vi "I2CConfigure.vi"(7 "Address Type (7-bit)":enum16{"7-bit", "10-bit"}(ring), 8 "error in (no error)":errorcluster caption="ErrorIn", 9 "Clock Rate":u32, 10 "IICSlaveAddress":u16, 11 "FPGA VI引用输入":refnum<k20>) -> (0 "error out":errorcluster caption="ErrorOut", 3 "FPGA VI引用输出":refnum<k20>)   [LabVIEW 2015]
uses:
  <vilib>/Utility/error.llb/Error Cluster From Error Code.vi
  <vilib>/rvi/errors/niLvFpgaAdjustHostInterfaceError.vi
  <vilib>/rvi/interface/nirviReadWriteControl/nirviReadWriteControl.xnode
  IEDriver/IEDriver/SPIandI2C/FPGA/Library/IP SPI&I2C.lvlib
  NiFpgaLv.dll
  <vilib>/rvi/interface/Simulation/niFpgaSimulationCallBeginRW.vi
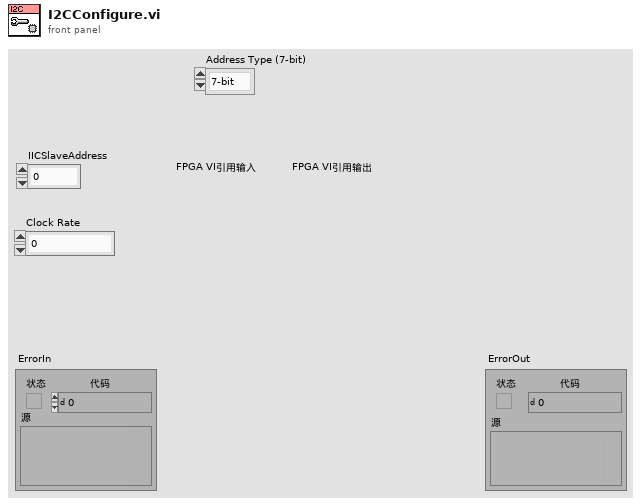
[diagram p1: front panel]
types:
  T1 = cluster{"Address Type (7-bit)":enum16{"7-bit", "10-bit"}, "IICSlaveAddress":u16, "I2C Parameters":cluster{"Clock Divider":u32}}
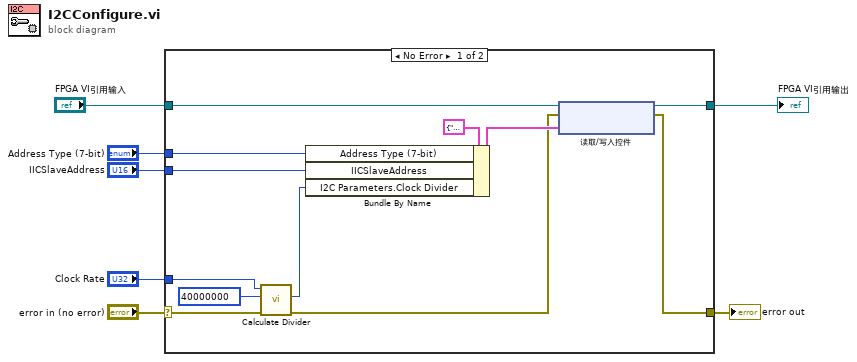
[diagram p0: block diagram]
diagram:
  n1 = case shown="No Error" "error in (no error)" {
    selector: "error in (no error)" -> [w18 w21]
    tunnel: "FPGA VI引用输入" -> [w19 w20]
    tunnel: "Clock Rate" -> [w16 _]
    tunnel: "Address Type (7-bit)" -> [w13 _]
    tunnel: "IICSlaveAddress" -> [w12 _]
    tunnel: [w9 w21] -> w3
    tunnel: [w8 w20] -> w1
    frame No Error {
      n2 = call "Calculate Divider.vi"("error in"=w18, "FPGA Clock (Hz)"=u32 40000000 ("Clock Rate (Hz)"), "Clock Rate (Hz)"=w16) -> ("error out"=w10:errorcluster, "Clock Divider"=w11:u32)  [unwired: 6 in, 1 out]
      n3 = Bundle By Name(cluster=T1 {"Address Type (7-bit)"=enum."7-bit", "IICSlaveAddress"=0, "I2C Parameters"={"Clock Divider"=0}} ("IICParameters"), "Address Type (7-bit)"=w13, "IICSlaveAddress"=w12, "I2C Parameters.Clock Divider"=w11) -> (w14:T1)
      n4 = xnode "读取/写入控件"("FPGA VI Reference In"=w19, "error in"=w10, "IICParameters"=w14) -> ("FPGA VI Reference Out"=w8:refnum<k20>, "error out"=w9:errorcluster)
    }
    frame Error {
    }
  }
  "error out" <- w3
  "FPGA VI引用输出" <- w1
